vi "ArdnoGetValveNums.vi"() -> (3 "Array":i32[](array[numeric]))   [LabVIEW 2018, in "Arduino.lvlib"]
uses:
  Arduino.lvlib
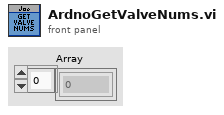
[diagram p1: front panel]
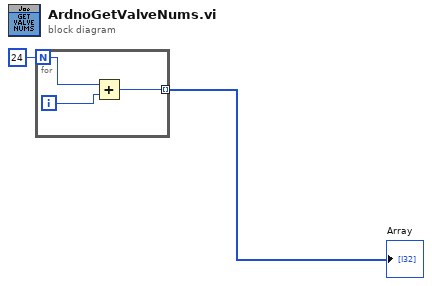
[diagram p0: block diagram]
diagram:
  n1 = for {
    N: 24 -> [w3]
    tunnel: [w4] -> w2 mode=indexing
    i -> [w5]
    n2 = Add(x=w3, y=w5) -> (x+y=w4:i32)
  }
  "Array" <- w2
